vi "ReadIOSettings.vi"   [LabVIEW 2020]
uses:
  <vilib>/Utility/sysdir.llb/System Directory Type.ctl
  global/SettingVariable.vi
  <vilib>/Utility/config.llb/Read Key (Boolean).vi
  <vilib>/Utility/config.llb/Read Key (String).vi
  <vilib>/Utility/config.llb/Read Key (I32).vi
  <vilib>/Utility/config.llb/Read Key (Double).vi
  <vilib>/Utility/config.llb/Read Key (U32).vi
  <vilib>/Utility/config.llb/Read Key (Path).vi
  <vilib>/Utility/config.llb/NI_LVConfig.lvlib
types:
  T1 = typedef "System Directory Type.ctl" = i32
  T2 = typedef "NI_LVConfig.lvlib/Config Data RefNum.ctl" = refnum<k1>
  T3 = cluster{"switch":bool, "voltage upper":i32, "voltage lower":i32, "physics upper":dbl, "physics lower":dbl, "input":u16, "log":bool}[]
  T4 = cluster{"switch":bool, "name":string, "voltage upper":i32, "voltage lower":i32, "physics upper":dbl, "physics lower":dbl, "scale":u16}[]
  T5 = cluster{"switch":bool, "name":string, "voltage upper":i32, "voltage lower":i32, "physics upper":dbl, "physics lower":dbl, "scale":u16}
  T6 = cluster{"switch":bool, "voltage upper":i32, "voltage lower":i32, "physics upper":dbl, "physics lower":dbl, "input":u16, "log":bool}
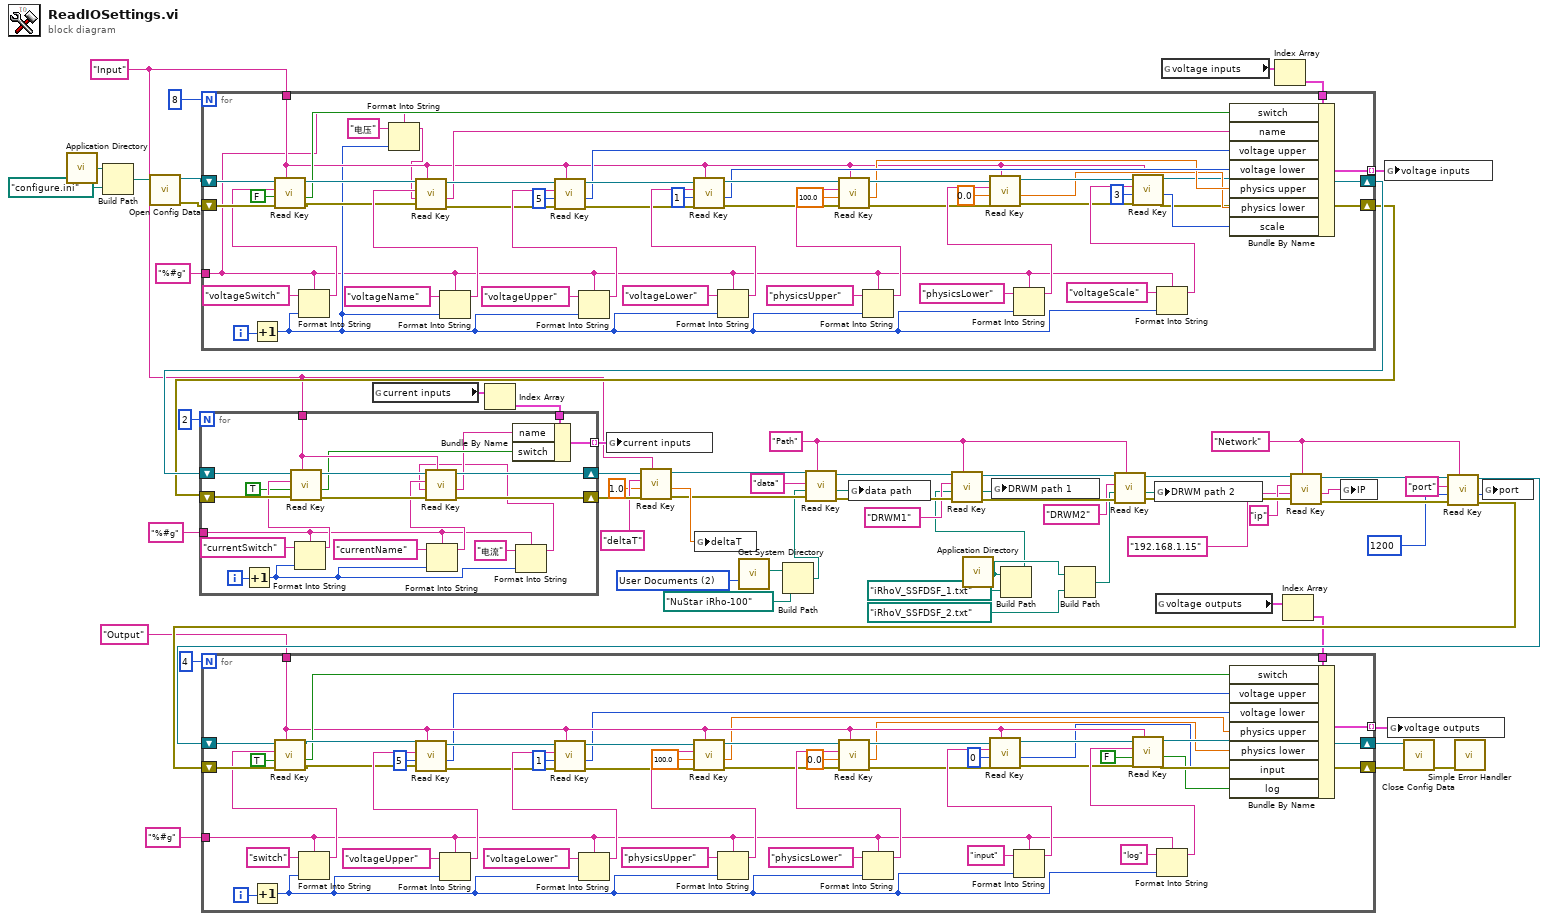
[diagram p0: block diagram]
diagram:
  w4 = T1 2 items=["User Home"=0, "User Desktop"=1, "User Documents"=2, "User Application Data"=3, "User Preferences"=4, "User Temporary"=5, "Public Documents"=6, "Public Application Data"=7, "Public Preferences"=8, "Public Cache"=13, "System Core Libraries"=9, "System Installed Libraries"=10, "Application Files"=11, "Boot Volume Root"=12] ("system directory type")
  w34 = "Network" ("section")
  w38 = "Path" ("section")
  w46 = "Input" ("section")
  n1 = call <vilib>:"Application Directory.vi"() -> ("Application Directory"=w67:path)
  n2 = Build Path(base path=w67, name or relative path=path "configure.ini") -> (appended path=w65:path)
  n3 = call <vilib>:"Open Config Data.vi"("configuration file path"=w65) -> ("error out"=w61:errorcluster, "refnum"=w62:T2)  [unwired: 8 in, 1 out]
  n4 = global read "SettingVariable.vi" "current inputs"() -> (w64:cluster{"name":string, "switch":bool}[])
  n5 = Index Array(array=w64) -> (element=w54:cluster{"name":string, "switch":bool})  [unwired: 1 in]
  n6 = call <vilib>:"Get System Directory.vi"("system directory type"=w4) -> ("system directory"=w3:path)  [unwired: 10 in]
  n7 = Build Path(base path=w3, name or relative path=path "NuStar iRho-100") -> (appended path=w1:path)
  n8 = call <vilib>:"Application Directory.vi"() -> ("Application Directory"=w7:path)
  n9 = Build Path(base path=w7, name or relative path=path "iRhoV_SSFDSF_1.txt") -> (appended path=w6:path)
  n10 = Build Path(base path=w7, name or relative path=path "iRhoV_SSFDSF_2.txt") -> (appended path=w5:path)
  n11 = global read "SettingVariable.vi" "voltage outputs"() -> (w20:T3)
  n12 = global read "SettingVariable.vi" "voltage inputs"() -> (w63:T4)
  n13 = Index Array(array=w63) -> (element=w60:T5)  [unwired: 1 in]
  n14 = for {
    N: 8 -> [_]
    tunnel: w46 -> [w80]
    tunnel: w60 -> [w89]
    tunnel: [w81] -> w59 mode=indexing
    shift-right: [w79] -> w56
    shift-left: w61 -> [w116]
    shift-right: [w78] -> w57
    shift-left: w62 -> [w117]
    tunnel: "%#g" ("format string") -> [w68]
    i -> [w118]
    n15 = Increment(x=w118) -> (x+1=w70:i32)
    n16 = Format Into String(format string=w68, initial string="voltageSwitch", w70) -> (resulting string=w114:string)  [unwired: 1 in, 1 out]
    n17 = call-poly <vilib>:"Read Key.vi"("section"=w80, "error in (no error)"=w116, "default value"=FALSE, "key"=w114, "refnum"=w117) -> ("error out"=w110:errorcluster, "value"=w87:bool, "refnum out"=w111:T2)  [unwired: 3 in, 1 out]
    n18 = Format Into String(format string=w68, initial string="电压", w70) -> (resulting string=w69:string)  [unwired: 1 in, 1 out]
    n19 = Format Into String(format string=w68, initial string="voltageName", w70) -> (resulting string=w113:string)  [unwired: 1 in, 1 out]
    n20 = call-poly <vilib>:"Read Key.vi"("section"=w80, "error in (no error)"=w110, "default value"=w69, "key"=w113, "refnum"=w111) -> ("error out"=w98:errorcluster, "value"=w86:string, "refnum out"=w99:T2)  [unwired: 3 in, 1 out]
    n21 = Format Into String(format string=w68, initial string="voltageUpper", w70) -> (resulting string=w108:string)  [unwired: 1 in, 1 out]
    n22 = call-poly <vilib>:"Read Key.vi"("section"=w80, "error in (no error)"=w98, "default value"=5, "key"=w108, "refnum"=w99) -> ("error out"=w96:errorcluster, "value"=w85:i32, "refnum out"=w97:T2)  [unwired: 3 in, 1 out]
    n23 = Format Into String(format string=w68, initial string="voltageLower", w70) -> (resulting string=w107:string)  [unwired: 1 in, 1 out]
    n24 = call-poly <vilib>:"Read Key.vi"("section"=w80, "error in (no error)"=w96, "default value"=1, "key"=w107, "refnum"=w97) -> ("error out"=w95:errorcluster, "value"=w84:i32, "refnum out"=w94:T2)  [unwired: 3 in, 1 out]
    n25 = Format Into String(format string=w68, initial string="physicsUpper", w70) -> (resulting string=w104:string)  [unwired: 1 in, 1 out]
    n26 = call-poly <vilib>:"Read Key.vi"("section"=w80, "error in (no error)"=w95, "default value"=100.0, "key"=w104, "refnum"=w94) -> ("error out"=w92:errorcluster, "value"=w83:dbl, "refnum out"=w93:T2)  [unwired: 3 in, 1 out]
    n27 = Format Into String(format string=w68, initial string="physicsLower", w70) -> (resulting string=w103:string)  [unwired: 1 in, 1 out]
    n28 = call-poly <vilib>:"Read Key.vi"("section"=w80, "error in (no error)"=w92, "default value"=0.0, "key"=w103, "refnum"=w93) -> ("error out"=w90:errorcluster, "value"=w82:dbl, "refnum out"=w91:T2)  [unwired: 3 in, 1 out]
    n29 = Format Into String(format string=w68, initial string="voltageScale", w70) -> (resulting string=w100:string)  [unwired: 1 in, 1 out]
    n30 = call-poly <vilib>:"Read Key.vi"("section"=w80, "error in (no error)"=w90, "default value"=u32 3, "key"=w100, "refnum"=w91) -> ("error out"=w79:errorcluster, "value"=w88:u32, "refnum out"=w78:T2)  [unwired: 3 in, 1 out]
    n31 = Bundle By Name(cluster=w89, "switch"=w87, "name"=w86, "voltage upper"=w85, "voltage lower"=w84, "physics upper"=w83, "physics lower"=w82, "scale"=w88) -> (w81:T5)
  }
  n32 = for {
    N: 2 -> [_]
    tunnel: w46 -> [w139]
    shift-right: [w132] -> w52
    shift-left: w57 -> [w136]
    shift-right: [w131] -> w51
    shift-left: w56 -> [w135]
    tunnel: w54 -> [w130]
    tunnel: [w127] -> w53 mode=indexing
    tunnel: "%#g" ("format string") -> [w120]
    i -> [w134]
    n33 = Increment(x=w134) -> (x+1=w122:i32)
    n34 = Format Into String(format string=w120, initial string="currentSwitch", w122) -> (resulting string=w133:string)  [unwired: 1 in, 1 out]
    n35 = call-poly <vilib>:"Read Key.vi"("section"=w139, "error in (no error)"=w135, "default value"=TRUE, "key"=w133, "refnum"=w136) -> ("error out"=w138:errorcluster, "value"=w129:bool, "refnum out"=w137:T2)  [unwired: 3 in, 1 out]
    n36 = Format Into String(format string=w120, initial string="currentName", w122) -> (resulting string=w124:string)  [unwired: 1 in, 1 out]
    n37 = Format Into String(format string=w120, initial string="电流", w122) -> (resulting string=w119:string)  [unwired: 1 in, 1 out]
    n38 = call-poly <vilib>:"Read Key.vi"("section"=w139, "error in (no error)"=w138, "default value"=w119, "key"=w124, "refnum"=w137) -> ("error out"=w131:errorcluster, "value"=w128:string, "refnum out"=w132:T2)  [unwired: 3 in, 1 out]
    n39 = Bundle By Name(cluster=w130, "name"=w128, "switch"=w129) -> (w127:cluster{"name":string, "switch":bool})
  }
  n40 = global write "SettingVariable.vi" "current inputs"(w53) -> ()
  n41 = call-poly <vilib>:"Read Key.vi"("section"=w46, "error in (no error)"=w51, "default value"=1.0, "key"="deltaT", "refnum"=w52) -> ("error out"=w47:errorcluster, "value"=w49:dbl, "refnum out"=w48:T2)  [unwired: 3 in, 1 out]
  n42 = global write "SettingVariable.vi" "deltaT"(w49) -> ()
  n43 = call-poly <vilib>:"Read Key.vi"("section"=w38, "error in (no error)"=w47, "default value"=w1, "key"="data", "refnum"=w48) -> ("error out"=w42:errorcluster, "value"=w45:path, "refnum out"=w41:T2)  [unwired: 3 in, 1 out]
  n44 = global write "SettingVariable.vi" "data path"(w45) -> ()
  n45 = call-poly <vilib>:"Read Key.vi"("section"=w38, "error in (no error)"=w42, "default value"=w6, "key"="DRWM1", "refnum"=w41) -> ("error out"=w39:errorcluster, "value"=w44:path, "refnum out"=w40:T2)  [unwired: 3 in, 1 out]
  n46 = global write "SettingVariable.vi" "DRWM path 1"(w44) -> ()
  n47 = call-poly <vilib>:"Read Key.vi"("section"=w38, "error in (no error)"=w39, "default value"=w5, "key"="DRWM2", "refnum"=w40) -> ("error out"=w31:errorcluster, "value"=w43:path, "refnum out"=w32:T2)  [unwired: 3 in, 1 out]
  n48 = global write "SettingVariable.vi" "DRWM path 2"(w43) -> ()
  n49 = Index Array(array=w20) -> (element=w19:T6)  [unwired: 1 in]
  n50 = call-poly <vilib>:"Read Key.vi"("section"=w34, "error in (no error)"=w31, "default value"="192.168.1.15", "key"="ip", "refnum"=w32) -> ("error out"=w30:errorcluster, "value"=w28:string, "refnum out"=w33:T2)  [unwired: 3 in, 1 out]
  n51 = global write "SettingVariable.vi" "IP"(w28) -> ()
  n52 = global write "SettingVariable.vi" "voltage inputs"(w59) -> ()
  n53 = call-poly <vilib>:"Read Key.vi"("section"=w34, "error in (no error)"=w30, "default value"=u32 1200, "key"="port", "refnum"=w33) -> ("error out"=w21:errorcluster, "value"=w26:u32, "refnum out"=w22:T2)  [unwired: 3 in, 1 out]
  n54 = for {
    N: 4 -> [_]
    tunnel: "Output" ("section") -> [w156]
    tunnel: w19 -> [w160]
    tunnel: [w157] -> w16 mode=indexing
    shift-right: [w155] -> w23
    shift-left: w21 -> [w187]
    shift-right: [w154] -> w24
    shift-left: w22 -> [w188]
    tunnel: "%#g" ("format string") -> [w147]
    i -> [w189]
    n55 = Increment(x=w189) -> (x+1=w159:i32)
    n56 = Format Into String(format string=w147, initial string="switch", w159) -> (resulting string=w185:string)  [unwired: 1 in, 1 out]
    n57 = call-poly <vilib>:"Read Key.vi"("section"=w156, "error in (no error)"=w187, "default value"=TRUE, "key"=w185, "refnum"=w188) -> ("error out"=w181:errorcluster, "value"=w158:bool, "refnum out"=w182:T2)  [unwired: 3 in, 1 out]
    n58 = Format Into String(format string=w147, initial string="voltageUpper", w159) -> (resulting string=w184:string)  [unwired: 1 in, 1 out]
    n59 = call-poly <vilib>:"Read Key.vi"("section"=w156, "error in (no error)"=w181, "default value"=5, "key"=w184, "refnum"=w182) -> ("error out"=w169:errorcluster, "value"=w152:i32, "refnum out"=w170:T2)  [unwired: 3 in, 1 out]
    n60 = Format Into String(format string=w147, initial string="voltageLower", w159) -> (resulting string=w179:string)  [unwired: 1 in, 1 out]
    n61 = call-poly <vilib>:"Read Key.vi"("section"=w156, "error in (no error)"=w169, "default value"=1, "key"=w179, "refnum"=w170) -> ("error out"=w167:errorcluster, "value"=w151:i32, "refnum out"=w168:T2)  [unwired: 3 in, 1 out]
    n62 = Format Into String(format string=w147, initial string="physicsUpper", w159) -> (resulting string=w178:string)  [unwired: 1 in, 1 out]
    n63 = call-poly <vilib>:"Read Key.vi"("section"=w156, "error in (no error)"=w167, "default value"=100.0, "key"=w178, "refnum"=w168) -> ("error out"=w166:errorcluster, "value"=w150:dbl, "refnum out"=w165:T2)  [unwired: 3 in, 1 out]
    n64 = Format Into String(format string=w147, initial string="physicsLower", w159) -> (resulting string=w175:string)  [unwired: 1 in, 1 out]
    n65 = call-poly <vilib>:"Read Key.vi"("section"=w156, "error in (no error)"=w166, "default value"=0.0, "key"=w175, "refnum"=w165) -> ("error out"=w163:errorcluster, "value"=w149:dbl, "refnum out"=w164:T2)  [unwired: 3 in, 1 out]
    n66 = Format Into String(format string=w147, initial string="input", w159) -> (resulting string=w174:string)  [unwired: 1 in, 1 out]
    n67 = call-poly <vilib>:"Read Key.vi"("section"=w156, "error in (no error)"=w163, "default value"=u32 0, "key"=w174, "refnum"=w164) -> ("error out"=w161:errorcluster, "value"=w148:u32, "refnum out"=w162:T2)  [unwired: 3 in, 1 out]
    n68 = Format Into String(format string=w147, initial string="log", w159) -> (resulting string=w171:string)  [unwired: 1 in, 1 out]
    n69 = call-poly <vilib>:"Read Key.vi"("section"=w156, "error in (no error)"=w161, "default value"=FALSE, "key"=w171, "refnum"=w162) -> ("error out"=w155:errorcluster, "value"=w153:bool, "refnum out"=w154:T2)  [unwired: 3 in, 1 out]
    n70 = Bundle By Name(cluster=w160, "switch"=w158, "voltage upper"=w152, "voltage lower"=w151, "physics upper"=w150, "physics lower"=w149, "input"=w148, "log"=w153) -> (w157:T6)
  }
  n71 = global write "SettingVariable.vi" "voltage outputs"(w16) -> ()
  n72 = call <vilib>:"Close Config Data.vi"("error in (no error)"=w23, "refnum"=w24) -> ("error out"=w25:errorcluster)  [unwired: 8 in, 1 out]
  n73 = call <vilib>:"Simple Error Handler.vi"("error in (no error)"=w25) -> ()  [unwired: 1 in, 8 out]
  n74 = global write "SettingVariable.vi" "port"(w26) -> ()
